vi "AIT 664 Initialization VI.vi"(8 "error in (no error)":errorcluster, 10 "Custom XML":string, 11 "Device Item Ref in":T1 format="%.0x") -> (0 "error out":errorcluster, 3 "Device Item Ref out":T1 format="%.0x")   [LabVIEW 2015, in "AIT 664 Custom Device.lvlib"]
uses:
  AIT 664 Custom Device.lvlib
  <vilib>/NI Veristand/Custom Device API/Custom Device Item Ref.ctl
  Controls and Global/Global.vi
  <vilib>/NI Veristand/Custom Device API/Custom Device API.lvlib
  <vilib>/NI Veristand/Custom Device Tools/Custom Device Utility Library/Custom Device Utility Library.lvlib
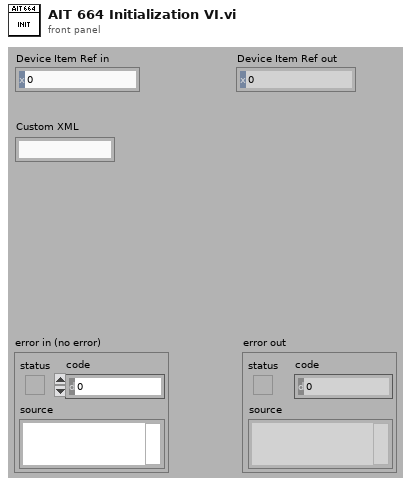
[diagram p1: front panel]
types:
  T1 = typedef "Custom Device API.lvlib/Custom Device Item Ref.ctl" = u64
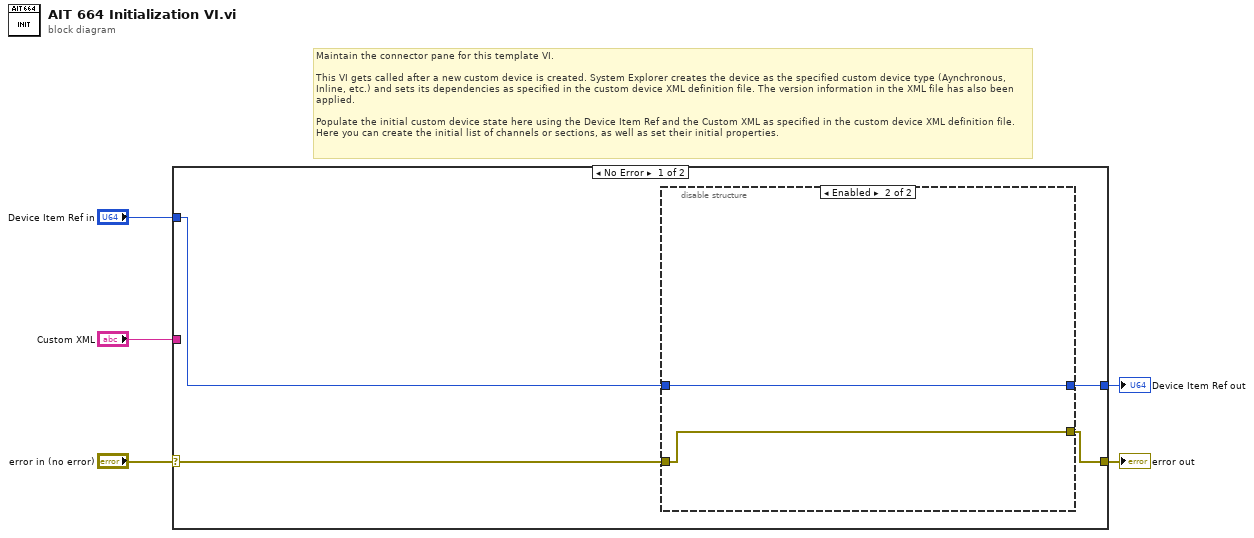
[diagram p0: block diagram]
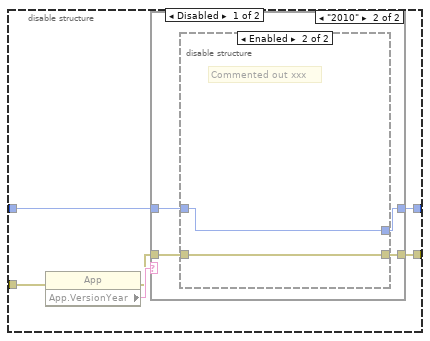
[diagram p2: hidden frame]
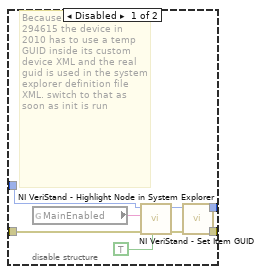
[diagram p4: hidden frame]
diagram:
  # "Maintain the connector pane for this template VI.\n\nThis VI gets called after a new custom device is created. System Explorer creates the device as the specified custom device type (Aynchronous, Inline, etc.) and sets its dependencies as specified in the custom device XML definition file. The version information in the XML file has also been applied.\n\nPopulate the initial custom device state here using the Device Item Ref and the Custom XML as specified in the custom device XML definition file. Here you can create the initial list of channels or sections, as well as set their initial properties."
  n1 = case shown="No Error" "error in (no error)" {
    selector: "error in (no error)" -> [w7 w35]
    tunnel: [w8 w34] -> w4
    tunnel: "Device Item Ref in" -> [w6 w34]
    tunnel: "Custom XML" -> [_ _]
    tunnel: [w9 w35] -> w1
    frame No Error {
      n2 = disable-structure shown="Enabled" {
        disable-tunnel: [w15 w33] -> w9
        disable-tunnel: [w14 w32] -> w8
        disable-tunnel: w7 -> [w11 w33]
        disable-tunnel: w6 -> [w10 w32]
        frame Disabled {
          n3 = property class="App"(error in=w11) -> (error out=w12:errorcluster, "App.VersionYear"=w13:string)  [unwired: 1 in, 1 out]
          n4 = case shown="\"2010\"" w13 {
            tunnel: w10 -> [w16 w21]
            tunnel: [w16 w20] -> w14
            tunnel: [w17 w18] -> w15
            tunnel: w12 -> [w17 w19]
            frame Default {
            }
            frame "2010" {
              n5 = disable-structure shown="Enabled" {
                disable-tunnel: w21 -> [w29 w31]
                disable-tunnel: [w25 w31] -> w20
                disable-tunnel: w19 -> [w23 w30]
                disable-tunnel: [w22 w30] -> w18
                frame Disabled {
                  # "Because of 2010 CAR 294615 the device in 2010 has to use a temp GUID inside its custom device XML and the real guid is used in the system explorer definition file XML. switch to that as soon as init is run"
                  n6 = global read "Global.vi" "MainEnabled"() -> (w28:string)
                  n7 = call <vilib>:"NI VeriStand - Set Item GUID.vi"("Refresh System Explorer Tree? (F)"=TRUE, "error in (no error)"=w23, "GUID"=w28, "Item Ref in"=w29) -> ("error out"=w27:errorcluster, "Item Ref out"=w26:T1)  [unwired: 6 in]
                  n8 = call <vilib>:"NI VeriStand - Highlight Node in System Explorer.vi"("error in (no error)"=w27, "Item Ref in"=w26) -> ("error out"=w22:errorcluster, "Node Ptr dup"=w25:T1)  [unwired: 8 in]
                }
                frame Enabled {
                  # "Commented out xxx"
                }
              }
            }
          }
        }
        frame Enabled {
        }
      }
    }
    frame Error {
    }
  }
  "error out" <- w1
  "Device Item Ref out" <- w4
